vi "sound_calibration_tdms.vi"() -> ()   [LabVIEW 2014]
uses:
  <vilib>/DAQmx/read.llb/DAQmx Read (Analog 1D Wfm NChan NSamp).vi
panel:
  out "起始":i32
  in  "保存时间":i32=5
  in  "创建新文件":bool=TRUE
  in  "数据文件保存路径":path=path "D:/压气机测试-2018-05-09/校准"
  in  "数据保存":bool
  out "波形图表":waveform(dbl)[](graph)
  in  "采样频率":dbl=50000.0 format="%0.2f"
  in  "stop":bool caption="停止"
  in  "通道":i32=1
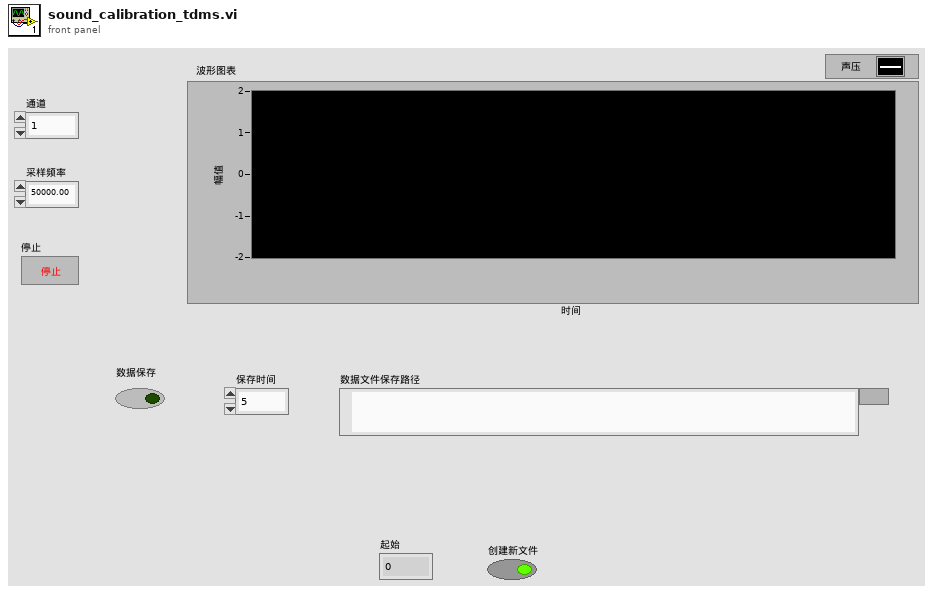
[diagram p1: front panel]
types:
  T1 = enum16{"open", "open or create", "create or replace", "create", "open (read-only)"}
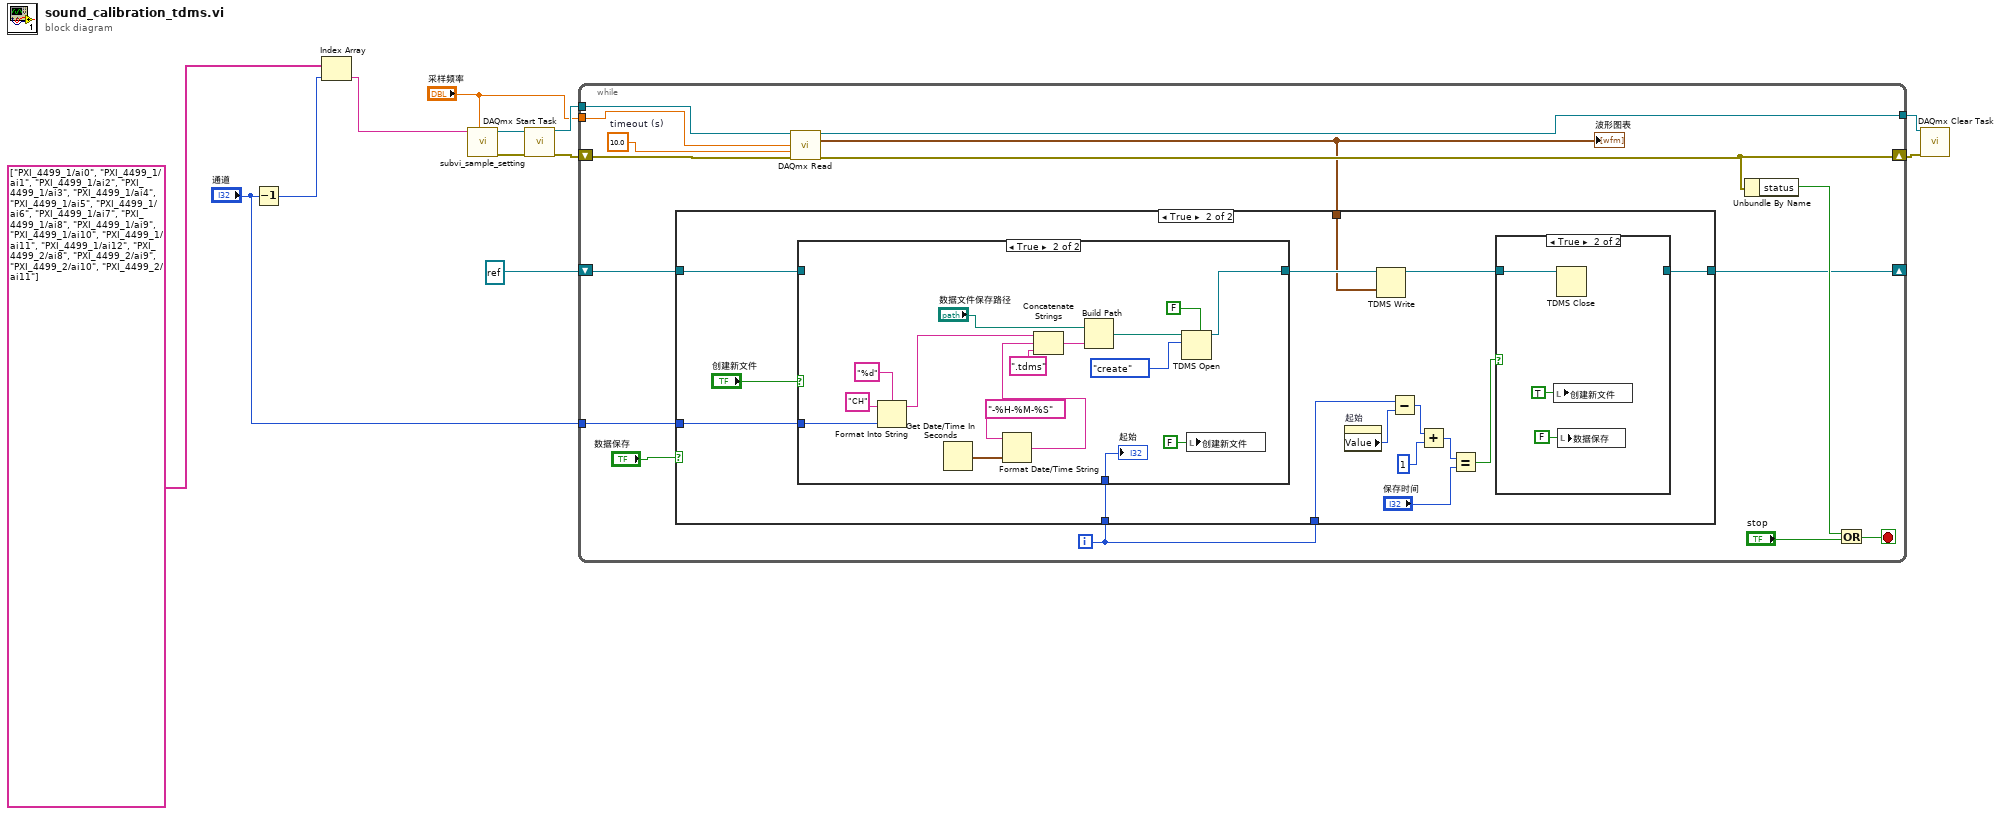
[diagram p0: block diagram]
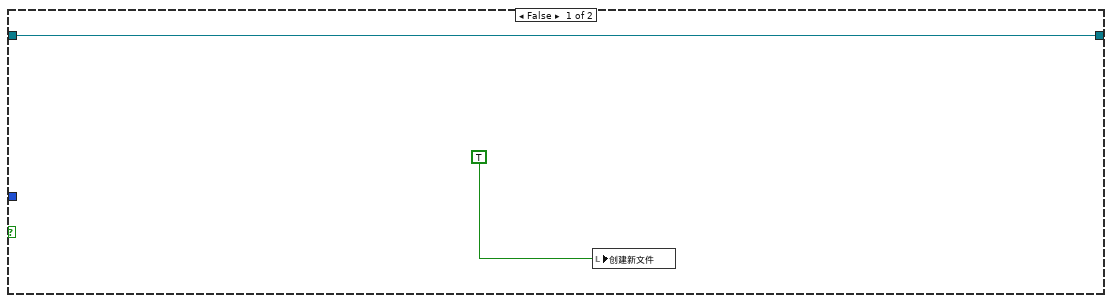
[diagram p2: hidden frame]
diagram:
  n1 = Decrement(x="通道") -> (x-1=w11:i32)
  n2 = Index Array(array=string[] ["PXI_4499_1/ai0", "PXI_4499_1/ai1", "PXI_4499_1/ai2", "PXI_4499_1/ai3", "PXI_4499_1/ai4", "PXI_4499_1/ai5", "PXI_4499_1/ai6", "PXI_4499_1/ai7", "PXI_4499_1/ai8", "PXI_4499_1/ai9", "PXI_4499_1/ai10", "PXI_4499_1/ai11", "PXI_4499_1/ai12", "PXI_4499_2/ai8", "PXI_4499_2/ai9", "PXI_4499_2/ai10", "PXI_4499_2/ai11"] ("添加的数组"), index=w11) -> (element=w4:string)
  n3 = call "subvi_sample_setting.vi"("采样频率"="采样频率", "physical channel"=w4) -> ("error out"=w6:errorcluster, "task out"=w5:refnum<k21>)  [unwired: 8 in]
  n4 = call <vilib>:"DAQmx Start Task.vi"("task/channels in"=w5, "error in"=w6) -> ("task out"=w10:refnum<k21>, "error out"=w9:errorcluster)  [unwired: 12 in]
  n5 = while "While循环" {
    tunnel: w10 -> [w27]
    tunnel: "采样频率" -> [w24]
    tunnel: [w25] -> w7
    shift-right: [w22] -> w8
    shift-left: w9 -> [w26]
    shift-right: [w16] -> _
    shift-left: refnum<k34> refnum ("tdms文件输出") -> [w17]
    tunnel: "通道" -> [w15]
    i -> [w13]
    stop <- w21 stop-if-true
    w19 = 10.0  # timeout (s)
    n6 = call-poly <vilib>:"DAQmx Read.vi"("task/channels in"=w27, "number of samples per channel"=w24, "timeout"=w19, "error in"=w26) -> ("task out"=w25:refnum<k21>, "data"=w14:waveform(dbl)[], "error out"=w22:errorcluster)  [unwired: 9 in]
    "波形图表" <- w14
    n7 = case shown="True" "数据保存" {
      tunnel: w17 -> [w29 w43]
      tunnel: [w29 w30] -> w16
      tunnel: w15 -> [_ w42]
      tunnel: w14 -> [_ w40]
      tunnel: w13 -> [_ w39]
      tunnel: w13 -> [_ w34]
      frame False {
        n8 = local write "创建新文件"(TRUE ("创建新文件")) -> ()
      }
      frame True {
        n9 = case shown="True" "创建新文件" {
          tunnel: w43 -> [w49 _]
          tunnel: [w49 w52] -> w41
          tunnel: w42 -> [_ w63]
          tunnel: w39 -> [_ w50]
          frame False {
          }
          frame True {
            n10 = Format Into String(format string="%d" ("格式字符串"), initial string="CH" ("初始字符串"), w63) -> (resulting string=w59:string)  [unwired: 1 in, 1 out]
            n11 = Get Date/Time In Seconds() -> (seconds since 1Jan1904=w61:timestamp)
            n12 = Format Date/Time String(time format string (%c)="-%H-%M-%S" ("时间格式字符串(%c)"), seconds (now)=w61) -> (date/time string=w58:string)  [unwired: 1 out]
            n13 = Concatenate Strings(w59, w58, ".tdms") -> (w60:string)
            n14 = Build Path(base path="数据文件保存路径", name or relative path=w60) -> (appended path=w55:path)
            n15 = TDMS Open(5:FALSE ("创建索引文件？(T)"), 10:T1."create" ("操作(0:open)"), 11:w55) -> (3:w52:refnum<k34>)  [unwired: 4 in, 1 out]
            n16 = local write "创建新文件"(FALSE ("创建新文件")) -> ()
            "起始" <- w50
          }
        }
        n17 = property on="起始" class="DigNum (strict)"() -> ("Value"=w35:i32)  [unwired: 2 in, 2 out]
        n18 = TDMS Write(0:w41, 9:w40) -> (4:w31:refnum<k34>)  [unwired: 4 in, 3 out]
        n19 = Subtract(x=w34, y=w35) -> (x-y=w38:i32)
        n20 = Add(x=w38, y=1) -> (x+y=w36:i32)
        n21 = Equal?(x=w36, y="保存时间") -> (x = y?=w32:bool)
        n22 = case shown="True" w32 {
          tunnel: w31 -> [w45 w48]
          tunnel: [w45 _] -> w30
          frame False {
          }
          frame True {
            n23 = local write "创建新文件"(TRUE ("创建新文件")) -> ()
            n24 = TDMS Close(11:w48) -> ()  [unwired: 1 in, 2 out]
            n25 = local write "数据保存"(FALSE ("数据保存")) -> ()
          }
        }
      }
    }
    n26 = Unbundle By Name(w22) -> ("status"=w23:bool)
    n27 = Or(x=w23, y="stop") -> (x .or. y?=w21:bool)
  }
  n28 = call <vilib>:"DAQmx Clear Task.vi"("task in"=w7, "error in"=w8) -> ()  [unwired: 13 in, 1 out]
